vi "Image Process mk1.vi"(3 "error out 2":errorcluster, 4 "IMAQ USB Session Out 2":T1, 5 "New Image":T2) -> (0 "error out":errorcluster, 1 "Image Out":T2, 2 "IMAQ USB Session Out":T1)   [LabVIEW 2011]
uses:
  <vilib>/vision/Image Controls.llb/IMAQ Image.ctl
  <vilib>/imaqUSB/imaqUSB.llb/IMAQ USB.ctl
  <vilib>/vision/NI_Vision_Development_Module.lvlib
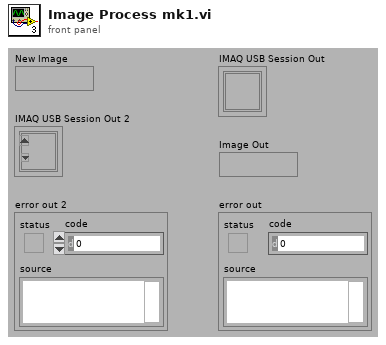
[diagram p1: front panel]
types:
  T1 = typedef "IMAQ USB.ctl" = refnum<k1>
  T2 = typedef "IMAQ Image.ctl" = refnum<image>
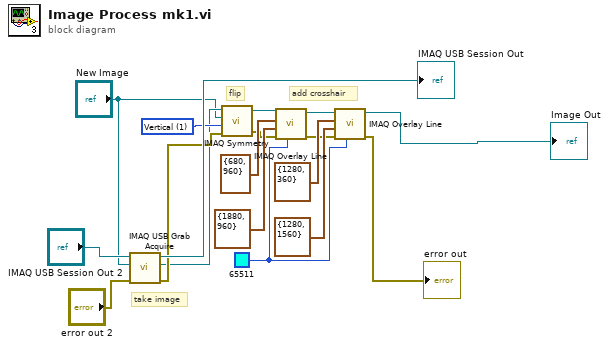
[diagram p0: block diagram]
diagram:
  w7 = u32 1 items=["Horizontal", "Vertical", "Central", "1st Diagonal", "2nd Diagonal"] ("Type of Symmetry")
  w18 = u32 65511 ("Color")
  # "add crosshair"
  # "flip"
  # "take image"
  n1 = call <vilib>:"IMAQ USB Grab Acquire.vi"("error in (no error)"="error out 2", "Image in"="New Image", "IMAQ USB Session In"="IMAQ USB Session Out 2") -> ("error out"=w5:errorcluster, "Image out"=w2:T2, "IMAQ USB Session Out"=→"IMAQ USB Session Out":T1)  [unwired: 6 out]
  n2 = call "IMAQ Symmetry"("error in (no error)"=w5, "Type of Symmetry"=w7, "Image Dst"="New Image", "Image Src"=w2) -> ("error out"=w3:errorcluster, "Image Dst Out"=w4:T2)  [unwired: 1 in]
  n3 = call "IMAQ Overlay Line"("Color"=w18, "error in (no error)"=w3, "End Point"=cluster{"X":i32, "Y":i32} {"X"=1880, "Y"=960}, "Start Point"=cluster{"X":i32, "Y":i32} {"X"=680, "Y"=960}, "Image"=w4) -> ("error out"=w9:errorcluster, "Image Out"=w17:T2)  [unwired: 1 in, 4 out]
  n4 = call "IMAQ Overlay Line"("Color"=w18, "error in (no error)"=w9, "End Point"=cluster{"X":i32, "Y":i32} {"X"=1280, "Y"=1560}, "Start Point"=cluster{"X":i32, "Y":i32} {"X"=1280, "Y"=360}, "Image"=w17) -> ("error out"=→"error out":errorcluster, "Image Out"=→"Image Out":T2)  [unwired: 1 in, 4 out]
